vi "Simulation Settings from ini.vi"(7 "Section":string, 8 "error in (no error)":errorcluster, 11 "Simulation Settings In":T1) -> (0 "error out":errorcluster, 3 "Simulation Settings Out":T1, 5 "All Tags Exists?":bool)   [LabVIEW 2013]
doc: "Loads the TCP port being used for listening for incoming connections."
uses:
  Simulation/Simulation Settings Cluster.ctl
  Simulation Enum Keys.ctl
  Common/File IO/INI/Read write mode.ctl
  Common/File IO/INI/INI Read write bool.vi
  Common/File IO/INI/INI Read write path.vi
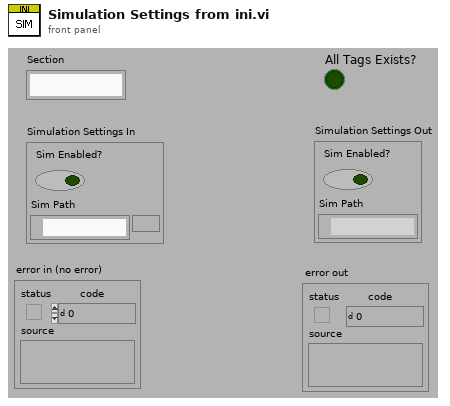
[diagram p1: front panel]
types:
  T1 = typedef "Simulation Settings Cluster.ctl" = cluster{"Sim Enabled?":bool, "Sim Path":path}
  T2 = typedef "Simulation Enum Keys.ctl" = enum16{"Enabled", "Path"}
  T3 = typedef "Read write mode.ctl" = enum16{"Read", "Write"}
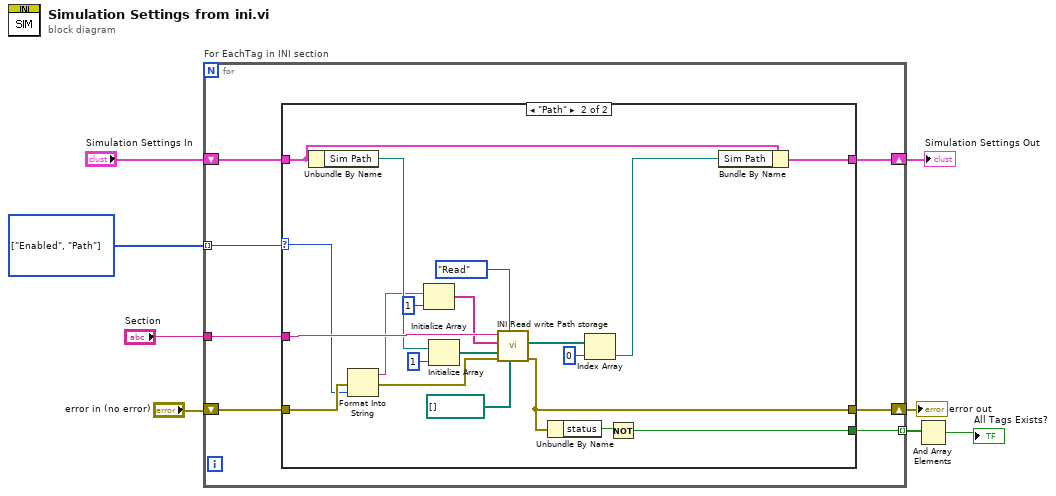
[diagram p0: block diagram]
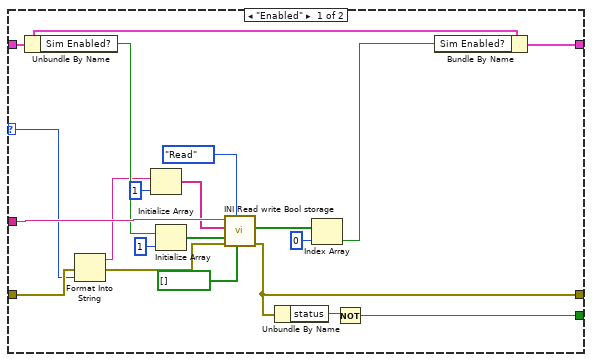
[diagram p2: hidden frame]
diagram:
  w8 = T2[] [enum."Enabled", enum."Path"] items=["Enabled", "Path"]
  n1 = for "For EachTag in INI section" {
    tunnel: "Section" -> [w15]
    tunnel: w8 -> [w14] mode=indexing
    shift-right: [w10] -> w6
    shift-left: "error in (no error)" -> [w12]
    shift-right: [w9] -> w1
    shift-left: "Simulation Settings In" -> [w13]
    tunnel: [w11] -> w4 mode=indexing
    n2 = case shown="\"Path\"" w14 {
      selector: w14 -> [w30 w50]
      tunnel: w15 -> [w34 w54]
      tunnel: w13 -> [w32 w52]
      tunnel: w12 -> [w31 w51]
      tunnel: [w35 w55] -> w10
      tunnel: [w17 w38] -> w11
      tunnel: [w33 w53] -> w9
      frame "Enabled" {
        n3 = Unbundle By Name(w32) -> ("Sim Enabled?"=w28:bool)
        n4 = Format Into String(error in=w31, w30) -> (resulting string=w25:string, error out=w18:errorcluster)  [unwired: 2 in]
        n5 = Initialize Array(w25, 1 ("dimension size")) -> (w23:string[])
        n6 = Initialize Array(w28, 1 ("dimension size")) -> (w26:bool[])
        n7 = call "INI Read write Bool storage.vi"("Values to write"=bool[] [], "Read/Write mode"=Read_write_mode."Read", "error in"=w18, "Defaults"=w26, "keys"=w23, "section"=w34) -> ("error out"=w35:errorcluster, "Values"=w22:bool[])  [unwired: 4 in]
        n8 = Unbundle By Name(w35) -> ("status"=w19:bool)
        n9 = Index Array(array=w22, index=0) -> (element=w20:bool)
        n10 = Not(x=w19) -> (.not. x?=w17:bool)
        n11 = Bundle By Name(cluster=w32, "Sim Enabled?"=w20) -> (w33:T1)
      }
      frame "Path" {
        n12 = Unbundle By Name(w52) -> ("Sim Path"=w48:path)
        n13 = Format Into String(error in=w51, w50) -> (resulting string=w46:string, error out=w39:errorcluster)  [unwired: 2 in]
        n14 = Initialize Array(w46, 1 ("dimension size")) -> (w44:string[])
        n15 = Initialize Array(w48, 1 ("dimension size")) -> (w36:path[])
        n16 = call "INI Read write Path storage.vi"("Values to write"=path[] [], "Read/Write mode"=Read_write_mode."Read", "error in"=w39, "Defaults"=w36, "keys"=w44, "section"=w54) -> ("error out"=w55:errorcluster, "Values"=w43:path[])  [unwired: 4 in]
        n17 = Unbundle By Name(w55) -> ("status"=w40:bool)
        n18 = Index Array(array=w43, index=0) -> (element=w41:path)
        n19 = Not(x=w40) -> (.not. x?=w38:bool)
        n20 = Bundle By Name(cluster=w52, "Sim Path"=w41) -> (w53:T1)
      }
    }
  }
  "error out" <- w6
  "Simulation Settings Out" <- w1
  n21 = And Array Elements(Boolean array=w4) -> (logical AND=→"All Tags Exists?":bool)
